vi "acquire.vi"(6 "Current Measurement":u32, 7 "Current Iteration":u32, 8 "error in (no error)":errorcluster, 10 "ExperimentVariables (in)":refnum<class "ExperimentVariables.lvclass">, 11 "Hamamatsu_C9100-13 in":refnum<class "Hamamatsu_C9100-13.lvclass">) -> (0 "error out":errorcluster, 1 "Array of ROI sums":dbl[][](array[numeric]), 2 "ExperimentVariables":refnum<class "ExperimentVariables.lvclass">, 3 "Hamamatsu_C9100-13 out":refnum<class "Hamamatsu_C9100-13.lvclass">, 5 "Image Array":T1[](array[plugin-control]))   [LabVIEW 2013]
uses:
  Hamamatsu_C9100-13.lvclass
  ExperimentVariables/ExperimentVariables.lvclass
  Camera.lvclass
panel:
  out "x-y":i32
  out "New Data?":bool
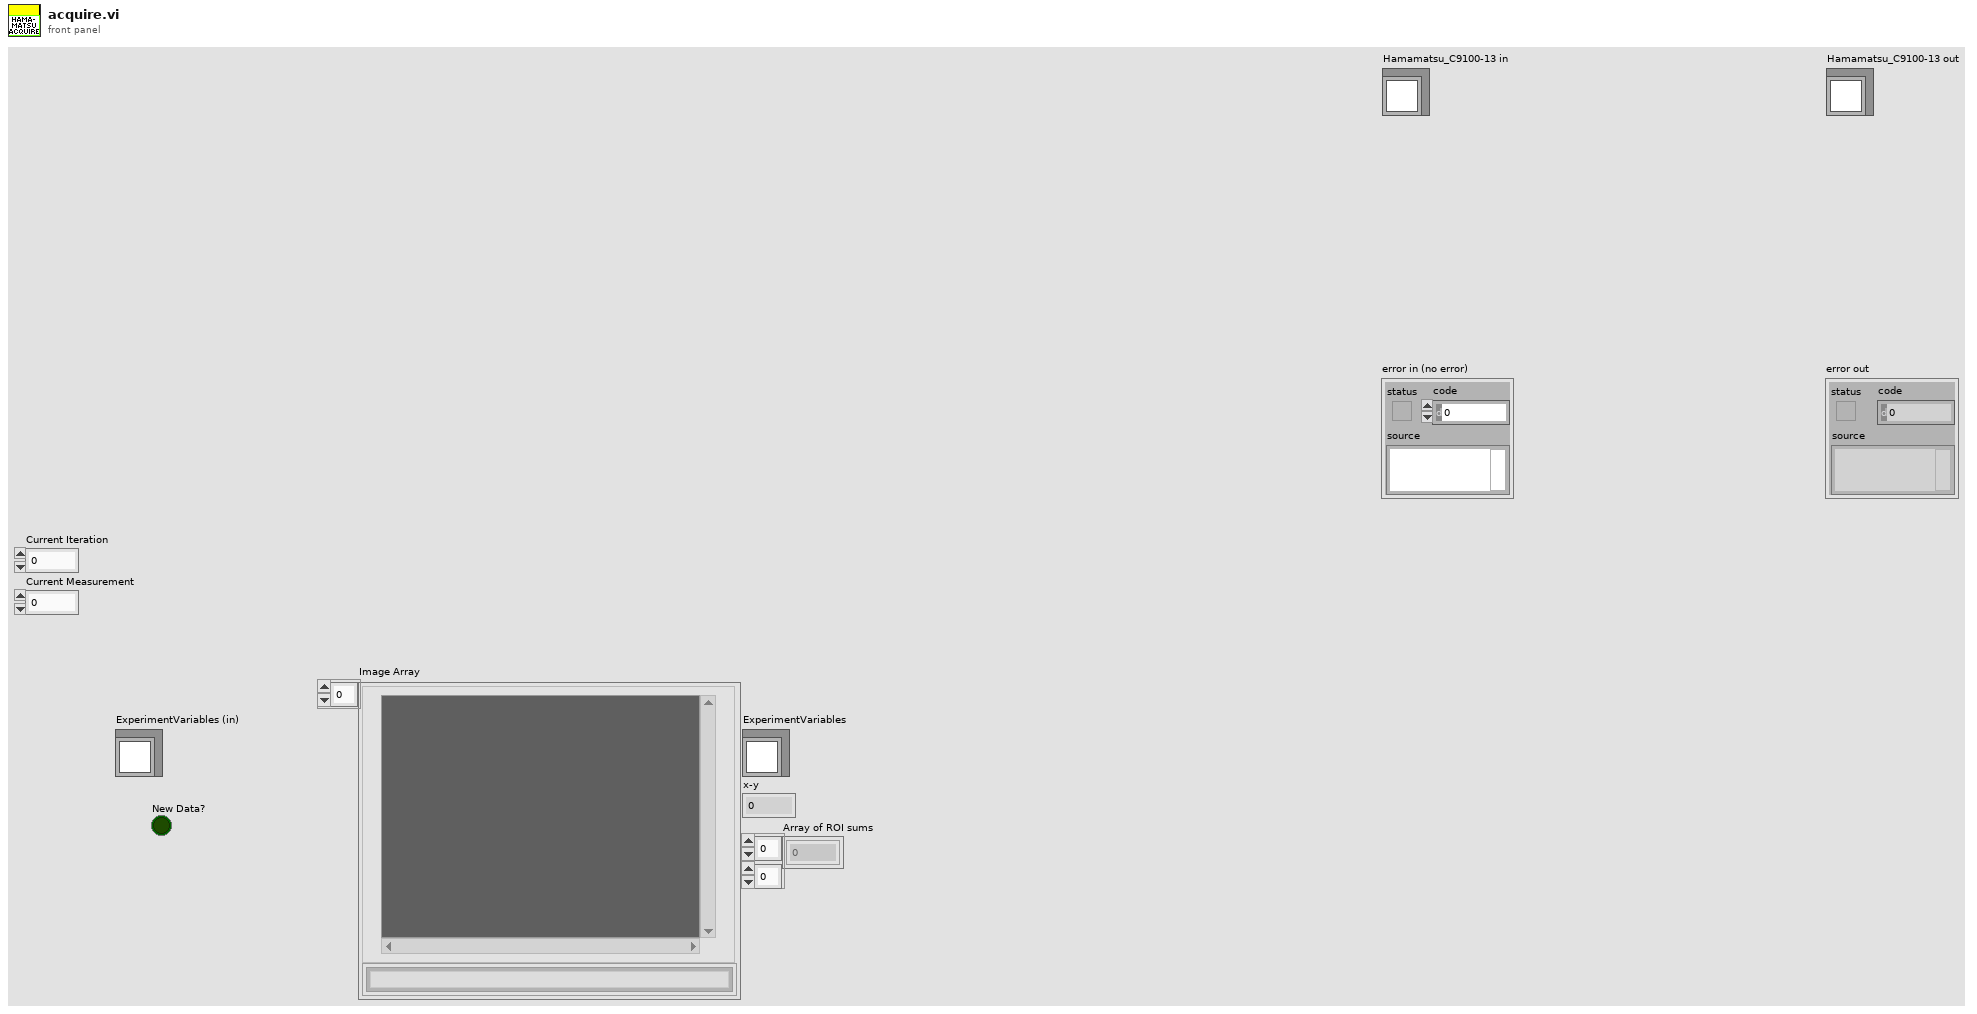
[diagram p1: front panel]
types:
  T1 = typedef "IMAQ Image.ctl" = refnum<image>
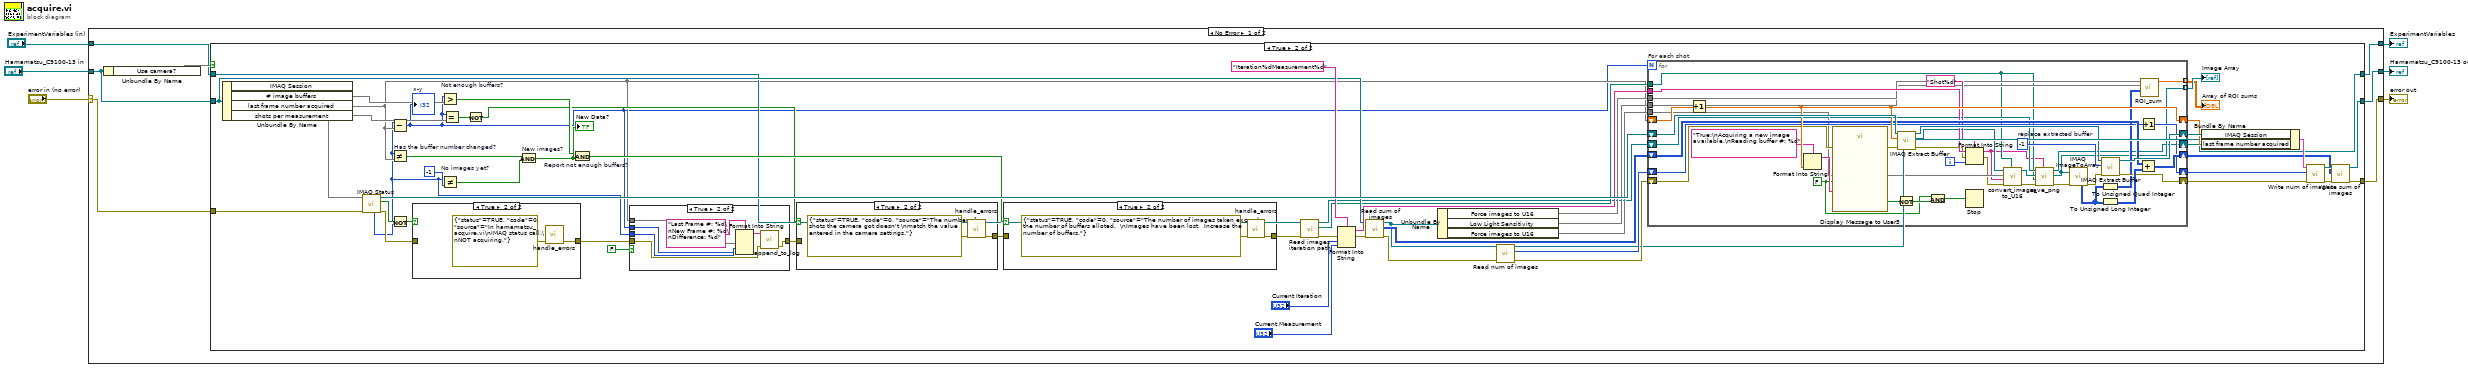
[diagram p0: block diagram]
diagram:
  n1 = case shown="No Error" "error in (no error)" {
    selector: "error in (no error)" -> [w13 w133]
    tunnel: [w12 w133] -> w5
    tunnel: [w9 w132] -> w3
    tunnel: "Hamamatsu_C9100-13 in" -> [w10 w132]
    tunnel: "ExperimentVariables (in)" -> [w8 w131]
    tunnel: [w7 w131] -> w1
    frame No Error {
      n2 = Unbundle By Name(w10) -> ("Use camera?"=w11)
      n3 = case shown="True" w11 {
        tunnel: w13 -> [w16 w64]
        tunnel: [w16 w51] -> w12
        tunnel: w8 -> [w15 w36]
        tunnel: [w15 w34] -> w7
        tunnel: w10 -> [w14 w49]
        tunnel: [w14 w54] -> w9
        frame False {
        }
        frame True {
          n4 = Unbundle By Name(w49) -> ("IMAQ Session"=w61, "# image buffers"=w60, "last frame number acquired"=w22, "shots per measurement"=w32)
          n5 = call <vilib>:"IMAQ Status.vi"("error in (no error)"=w64, "IMAQ Session In"=w61) -> ("error out"=w26:errorcluster, "Acquiring?"=w65:bool, "IMAQ Session Out"=w71:refnum<k11>, "Last Valid Buffer Number"=w21:i32)  [unwired: 5 in, 1 out]
          n6 = Subtract(x=w21, y=w22) -> (x-y=w20:i32)
          "x-y" <- w20
          n7 = Not Equal? "Has the buffer number changed?"(x=w21, y=w22) -> (x != y?=w67:bool)
          n8 = Not(x=w65) -> (.not. x?=w27:bool)
          n9 = case shown="True" w27 {
            tunnel: [w81 w83] -> w24
            tunnel: w26 -> [w81 _]
            frame False {
            }
            frame True {
              n10 = call "handle_errors.vi"("error in (no error)"=errorcluster {"status"=TRUE, "code"=0, "source"="In hamamatsu_acquire.vi\nIMAQ status call.\nNOT acquiring."} ("error constant")) -> ("error out"=w83:errorcluster)  [unwired: 10 in]
            }
          }
          n11 = Greater? "Not enough buffers?"(x=w20, y=w60) -> (0:w69:bool)
          n12 = Not Equal? "No images yet?"(x=w21, y=-1) -> (x != y?=w66:bool)
          n13 = Equal?(x=w20, y=w32) -> (x = y?=w31:bool)
          n14 = Not(x=w31) -> (.not. x?=w28:bool)
          n15 = Compound Arithmetic op=AND "New images?"(w67, w66) -> (w72:bool)
          "New Data?" <- w72
          n16 = And "Report not enough buffers?"(x=w69, y=w72) -> (x .and. y?=w68:bool)
          n17 = case shown="True" FALSE ("Enable") {
            tunnel: [w73 w80] -> w23
            tunnel: w24 -> [w73 w79]
            tunnel: w22 -> [_ w76]
            tunnel: w21 -> [_ w75]
            tunnel: w20 -> [_ w74]
            frame False {
            }
            frame True {
              n18 = Format Into String(format string="Last Frame #: %d\nNew Frame #: %d\nDifference: %d", w76, w75, w74) -> (resulting string=w77:string)  [unwired: 2 in, 1 out]
              n19 = call "append_to_log.vi"("error in"=w79, "string"=w77) -> ("error out"=w80:errorcluster)  [unwired: 9 in]
            }
          }
          n20 = case shown="True" w28 {
            tunnel: [w84 w86] -> w29
            tunnel: w23 -> [w84 _]
            frame False {
            }
            frame True {
              n21 = call "handle_errors.vi"("error in (no error)"=errorcluster {"status"=TRUE, "code"=0, "source"="The number of shots the camera got doesn't \nmatch the value entered in the camera settings."} ("error constant")) -> ("error out"=w86:errorcluster)  [unwired: 10 in]
            }
          }
          n22 = case shown="True" w68 {
            tunnel: w29 -> [w128 _]
            tunnel: [w128 w130] -> w37
            frame False {
            }
            frame True {
              n23 = call "handle_errors.vi"("error in (no error)"=errorcluster {"status"=TRUE, "code"=0, "source"="The number of images taken exceeds the number of buffers alloted.  \nImages have been lost.  Increase the number of buffers."} ("error constant")) -> ("error out"=w130:errorcluster)  [unwired: 10 in]
            }
          }
          n24 = call-dynamic "Read images iteration path.vi"("error in (no error)"=w37, "ExperimentVariables in"=w36) -> ("error out"=w17:errorcluster, "images iteration path"=w35:path, "ExperimentVariables out"=w30:refnum<class "ExperimentVariables.lvclass">)  [unwired: 7 in]
          n25 = Format Into String(format string="Iteration%dMeasurement%d", error in=w17, "Current Iteration", "Current Measurement") -> (resulting string=w62:string, error out=w48:errorcluster)  [unwired: 1 in]
          n26 = call-dynamic "Read sum of images.vi"("error in (no error)"=w48, "Camera in"=w49) -> ("error out"=w41:errorcluster, "sum of images"=w50:u32[][], "Camera out"=w39:refnum<class "Hamamatsu_C9100-13.lvclass">)  [unwired: 7 in]
          n27 = Unbundle By Name(w39) -> ("Force images to U16"=w45, "Low Light Sensitivity"=w44, "Force images to U16"=w33)
          n28 = call-dynamic "Read num of images.vi"("error in (no error)"=w41, "Camera in"=w39) -> ("error out"=w40:errorcluster, "# of images"=w42:u32, "Camera out"=w38:refnum<class "Hamamatsu_C9100-13.lvclass">)  [unwired: 7 in]
          n29 = for "For each shot" {
            N: w20 -> [_]
            shift-right: [w124] -> w47
            shift-left: w22 -> [w127]
            shift-right: [w119] -> w59
            shift-left: w71 -> [w126]
            shift-right: [w107] -> w57
            shift-left: w40 -> [w115]
            tunnel: [w91] -> w46 mode=indexing
            shift-right: [w114] -> w53
            shift-left: w50 -> [w113]
            shift-right: [w110] -> w56
            shift-left: w42 -> [w111]
            tunnel: w35 -> [w88]
            tunnel: w62 -> [w106]
            tunnel: w45 -> [w102]
            tunnel: w44 -> [w101]
            tunnel: [w99] -> w43 mode=indexing
            shift-right: [w89] -> w34
            shift-left: w30 -> [w90]
            tunnel: w33 -> [w96]
            i -> [w104]
            w117 = FALSE ("Enable")
            w121 = -1  # replace extracted buffer
            n30 = Increment(x=w127) -> (x+1=w124:dbl)
            n31 = Format Into String(format string="True:\nAcquiring a new image available.\nReading buffer #: %d", w124) -> (resulting string=w122:string)  [unwired: 2 in, 1 out]
            n32 = call "Display Message to User3"("error in (no error)"=w115, "Enable"=w117, "Message"=w122) -> ("error out"=w109:errorcluster, "OK"=w125:bool)  [unwired: 7 in]
            n33 = Not(x=w125) -> (.not. x?=w118:bool)
            n34 = call <vilib>:"IMAQ Extract Buffer.vi"("error in (no error)"=w109, "Buffer to extract"=w124, "IMAQ Session In"=w126) -> ("error out"=w98:errorcluster, "Image Out"=w97:T1, "IMAQ Session Out"=w120:refnum<k11>)  [unwired: 3 in, 3 out]
            n35 = And(x=w117, y=w118) -> (x .and. y?=w116:bool)
            n36 = Format Into String(format string="Shot%d", initial string=w106, error in=w98, w104) -> (resulting string=w87:string, error out=w95:errorcluster)
            n37 = Stop(stop? (T)=w116) -> ()
            n38 = call "convert_image_to_U16.vi"("File Path"=w88, "error in (no error)"=w95, "Image Name"=w87, "Convert to U16?"=w96, "Image"=w97) -> ("error out"=w94:errorcluster, "Image Out"=w92:T1)  [unwired: 4 in, 1 out]
            n39 = call "save_png.vi"("shot name"=w87, "error in (no error)"=w94, "File Path"=w88, "Image In"=w92, "ExperimentVariables in"=w90) -> ("error out"=w93:errorcluster, "Image Out (duplicate)"=w91:T1, "ExperimentVariables out"=w89:refnum<class "ExperimentVariables.lvclass">)  [unwired: 4 in]
            n40 = call "IMAQ ImageToArray"("error in (no error)"=w93, "Image"=w91) -> ("Image Pixels (U16)"=w103:u16[][], "error out"=w108:errorcluster)  [unwired: 2 in, 3 out]
            n41 = To Unsigned Quad Integer(1:w103) -> (0:w100:u64[][])
            n42 = To Unsigned Long Integer(number=w103) -> (unsigned 32bit integer=w112:u32[][])
            n43 = call <vilib>:"IMAQ Extract Buffer.vi"("error in (no error)"=w108, "Buffer to extract"=w121, "IMAQ Session In"=w120) -> ("error out"=w107:errorcluster, "IMAQ Session Out"=w119:refnum<k11>)  [unwired: 3 in, 4 out]
            n44 = Add(x=w113, y=w112) -> (x+y=w114:u32[][])
            n45 = Increment(x=w111) -> (x+1=w110:u32)
            n46 = call "ROI_sum.vi"("unsigned 64bit integer"=w100, "Background Regions (Left, Top, Right, Bottom)"=w101, "Regions of Interest (Left, Top, Right, Bottom)"=w102) -> ("Array of ROI sums"=w99:dbl[])  [unwired: 8 in]
          }
          "Image Array" <- w46
          "Array of ROI sums" <- w43
          n47 = Bundle By Name(cluster=w38, "IMAQ Session"=w59, "last frame number acquired"=w47) -> (w58:cluster{})
          n48 = call-dynamic "Write num of images.vi"("error in (no error)"=w57, "# of images"=w56, "Camera in"=w58) -> ("error out"=w52:errorcluster, "Camera out"=w55:refnum<class "Camera.lvclass">)  [unwired: 7 in]
          n49 = call-dynamic "Write sum of images.vi"("error in (no error)"=w52, "sum of images"=w53, "Camera in"=w55) -> ("error out"=w51:errorcluster, "Camera out"=w54:refnum<class "Camera.lvclass">)  [unwired: 7 in]
        }
      }
    }
    frame Error {
    }
  }
  "error out" <- w5
  "Hamamatsu_C9100-13 out" <- w3
  "ExperimentVariables" <- w1
